vi "Find All Components.vi"(8 "error in (no error)":errorcluster, 11 "XML Doc Ref in":refnum<k20>) -> (0 "error out":errorcluster, 2 "Component Types":string[](array[string]), 3 "Nodes":refnum<k20>[](array[refnum]))   [LabVIEW 2020]
doc: "Finds all the Components defined for a single Board in the XML file while also returning their types and references to their component nodes."
uses:
  <resource>/objmgr/DOMUserDefRef.rc
  <vilib>/xml/NI_XML.lvlib
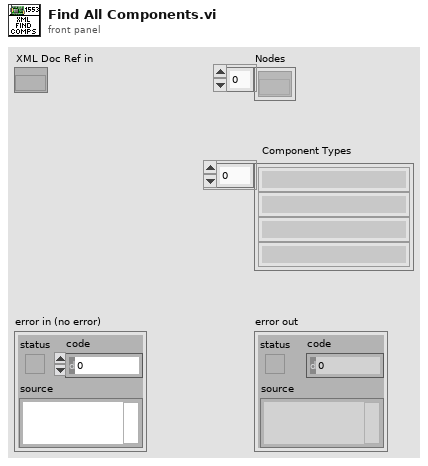
[diagram p1: front panel]
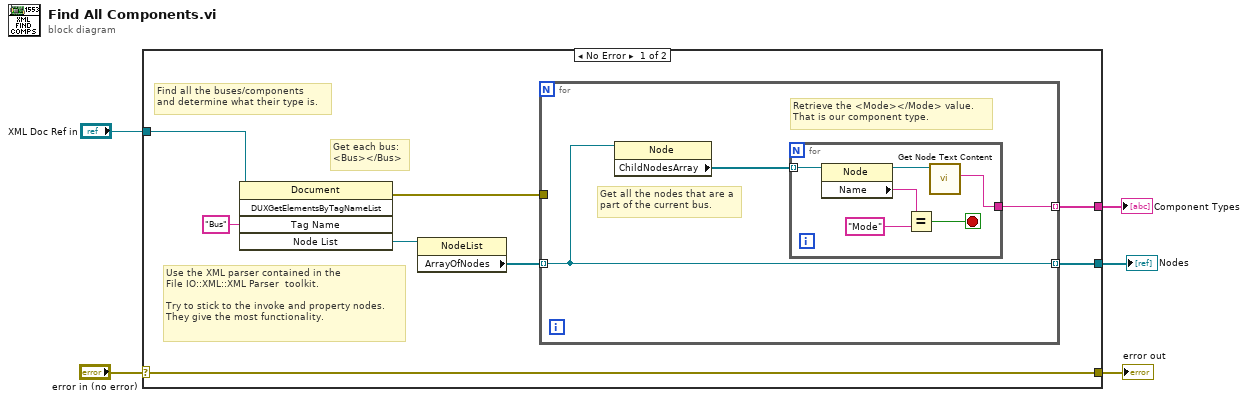
[diagram p0: block diagram]
diagram:
  n1 = case shown="No Error" "error in (no error)" {
    selector: "error in (no error)" -> [w13 w23]
    tunnel: [w13 w23] -> w4
    tunnel: "XML Doc Ref in" -> [w6 _]
    tunnel: [w11 _] -> w2
    tunnel: [w9 _] -> w1
    frame No Error {
      # "Get each bus:\n<Bus></Bus>"
      # "Find all the buses/components\nand determine what their type is."
      # "Use the XML parser contained in the\nFile IO::XML::XML Parser  toolkit.\n\nTry to stick to the invoke and property nodes.\nThey give the most functionality."
      n2 = invoke class="Document" method="DUXGetElementsByTagNameList"(reference=w6, "Tag Name"="Bus") -> (error out=w7:errorcluster, "Node List"=w12:refnum<k20>)  [unwired: 3 in, 3 out]
      n3 = property class="NodeList"(reference=w12) -> ("ArrayOfNodes"=w10:refnum<k20>[])  [unwired: 1 in, 2 out]
      n4 = for {
        tunnel: [w14] -> w11 mode=indexing
        tunnel: w10 -> [w14] mode=indexing
        tunnel: [w16] -> w9 mode=indexing
        tunnel: w7 -> [_]
        # "Retrieve the <Mode></Mode> value.\nThat is our component type."
        # "Get all the nodes that are a\npart of the current bus."
        n5 = property class="Node"(reference=w14) -> ("ChildNodesArray"=w15:refnum<k20>[])  [unwired: 1 in, 2 out]
        n6 = for {
          tunnel: w15 -> [w22] mode=indexing
          tunnel: [w17] -> w16
          stop <- w20 stop-if-true
          n7 = property class="Node"(reference=w22) -> (reference out=w18:refnum<k20>, "Name"=w19:string)  [unwired: 1 in, 1 out]
          n8 = Equal?(x=w19, y="Mode") -> (x = y?=w20:bool)
          n9 = call <vilib>:"Get Node Text Content.vi"("node in"=w18) -> ("node text"=w17:string)  [unwired: 8 in, 2 out]
        }
      }
    }
    frame Error {
    }
  }
  "error out" <- w4
  "Component Types" <- w1
  "Nodes" <- w2
